vi "_API_BINANCE_GET_USDT_FUTURES_TickSize.vi"(0 "BinanceAPI in":refnum<class "BinanceAPI_.lvclass">, 5 "TickSize":cluster{"symbol (eg. BTCUSDT)":string}, 11 "error in (no error)":errorcluster) -> (4 "BinanceAPI out":refnum<class "BinanceAPI_.lvclass">, 6 "tickSize":dbl format="%#.6f", 14 "Body":string, 15 "error out":errorcluster)   [LabVIEW 2022 SP3, in "BinanceAPI_.lvclass"]
doc: "https://binance-docs.github.io/apidocs/futures/en/#exchange-information\n\n<B>tickSize</B> -- minimal step of e.g. quantity in $$$ in price you sell your crypto. E.g. if is equal for Bitcoin 1 (one) you can buy bitcoins for 9999.0 dolars, 10000.0 dolars or 10001.0 dolars.s"
uses:
  BinanceAPI_.lvclass
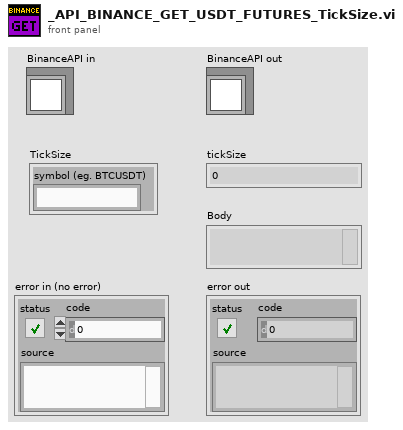
[diagram p1: front panel]
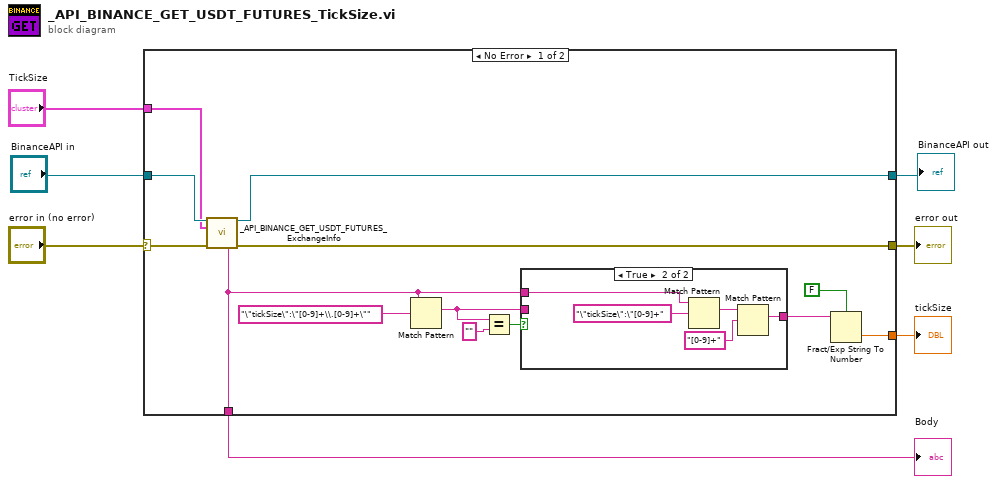
[diagram p0: block diagram]
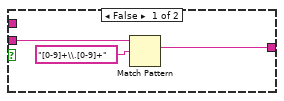
[diagram p2: hidden frame]
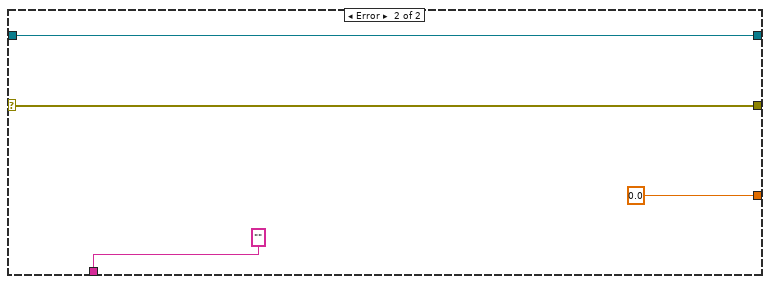
[diagram p3: hidden frame]
diagram:
  n1 = case shown="No Error" "error in (no error)" {
    selector: "error in (no error)" -> [w10 w31]
    tunnel: [w17 0.0] -> w7
    tunnel: [w15 w31] -> w6
    tunnel: [w14 w32] -> w1
    tunnel: "BinanceAPI in" -> [w13 w32]
    tunnel: "TickSize" -> [w8 _]
    tunnel: [w9 "" ("Body")] -> w3
    frame No Error {
      n2 = call "_API_BINANCE_GET_USDT_FUTURES_ExchangeInfo.vi"("BinanceAPI in"=w13, "exchangeInfo"=w8, "error in (no error)"=w10) -> ("BinanceAPI out"=w14:refnum<class "BinanceAPI_.lvclass">, "insideInfo"=w9:string, "error out"=w15:errorcluster)  [unwired: 8 in, 2 out]
      n3 = Match Pattern(string=w9, regular expression="\"tickSize\":\"[0-9]+\\.[0-9]+\"") -> (match substring=w19:string)  [unwired: 1 in, 3 out]
      n4 = Equal?(x=w19, y="" ("match substring")) -> (x = y?=w20:bool)
      n5 = case shown="True" w20 {
        tunnel: [w22 w24] -> w12
        tunnel: w19 -> [w21 _]
        tunnel: w9 -> [_ w27]
        frame False {
          n6 = Match Pattern(string=w21, regular expression="[0-9]+\\.[0-9]+") -> (match substring=w22:string)  [unwired: 1 in, 3 out]
        }
        frame True {
          n7 = Match Pattern(string=w27, regular expression="\"tickSize\":\"[0-9]+") -> (match substring=w25:string)  [unwired: 1 in, 3 out]
          n8 = Match Pattern(string=w25, regular expression="[0-9]+") -> (match substring=w24:string)  [unwired: 1 in, 3 out]
        }
      }
      n9 = Fract/Exp String To Number(use system decimal point (T)=FALSE, string=w12) -> (number=w17:dbl)  [unwired: 2 in, 1 out]
    }
    frame Error {
    }
  }
  "tickSize" <- w7
  "error out" <- w6
  "Body" <- w3
  "BinanceAPI out" <- w1
